vi "DSF.Shared.Configuration.Framework.Convert.From JSON Cluster.vi"(8 "error in (no error)":errorcluster, 10 "Framework Config (JSON)":T1, 11 "Framework Configuration in":refnum<class "DSF.Shared.Configuration.Framework.lvclass">) -> (0 "error out":errorcluster, 3 "Framework Configuration out":refnum<class "DSF.Shared.Configuration.Framework.lvclass">)   [LabVIEW 2017, in "DSF.Engine.lvlib" / "DSF.Shared.Configuration.Framework.lvclass"]
uses:
  DSF.Shared.Configuration.Framework.lvclass
  Typedefs/DELETE.DSF Framework Configuration.ctl
  Typedefs/DELETE.DSF Plugin Configuration.ctl
  DSF Configuration API/1.0.0/Public/Controls/DSF Timing Info.ctl
  Typedefs/DELETE.DSF Transfer Group Configuration.ctl
  Typedefs/DELETE.DSF.Shared.Refactor.Typedefs.JSON.Transfer Configuration.ctl
  DSF Configuration API/1.0.0/Public/Controls/DSF Byte Order.ctl
  Typedefs/DELETE.DSF.Shared.Refactor.Typedefs.JSON.Channel Array Configuration.ctl
  DSF Configuration API/1.0.0/Public/Controls/DSF Settings Info.ctl
  DSF.Shared.Configuration.Framework.lvclass/DSF.Shared.Configuration.Framework.ctl
  DSF.Engine.lvlib
  DSF Configuration API/1.0.0/DSF Configuration API.lvlib
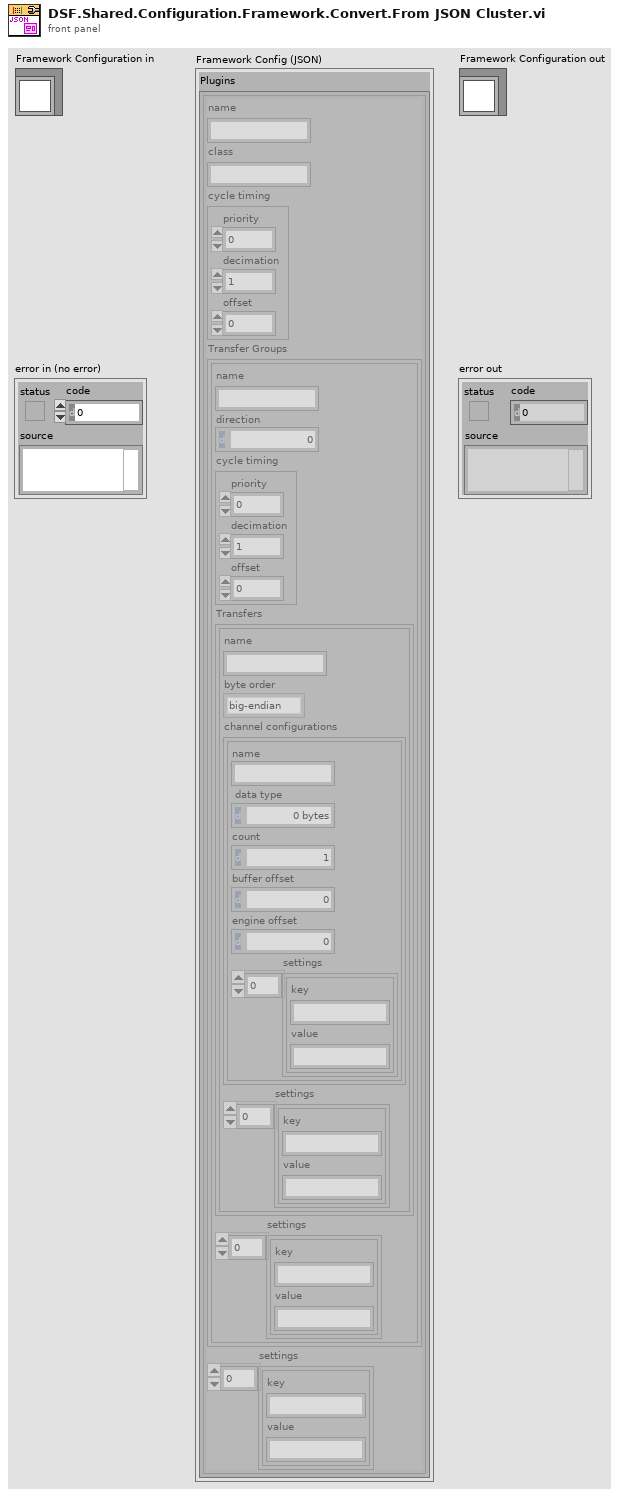
[diagram p1: front panel]
types:
  T1 = typedef "DSF.Engine.lvlib/DELETE.DSF Framework Configuration.ctl" = cluster{"Plugins":T2[]}
  T2 = typedef "DSF.Engine.lvlib/DELETE.DSF Plugin Configuration.ctl" = cluster{"name":string, "class":string, "cycle timing":T3, "Transfer Groups":T4[], "settings":T8}
  T3 = typedef "DSF Configuration API.lvlib/DSF Timing Info.ctl" = cluster{"priority":i32, "decimation":i32, "offset":i32}
  T4 = typedef "DSF.Engine.lvlib/DELETE.DSF Transfer Group Configuration.ctl" = cluster{"name":string, "direction":u8, "cycle timing":T3, "Transfers":T5[], "settings":T8}
  T5 = typedef "DSF.Engine.lvlib/DELETE.DSF.Shared.Refactor.Typedefs.JSON.Transfer Configuration.ctl" = cluster{"name":string, "byte order":T6, "channel configurations":T7[], "settings":T8}
  T6 = typedef "DSF Configuration API.lvlib/DSF Byte Order.ctl" = enum8{"big-endian", "little-endian"}
  T7 = typedef "DSF.Engine.lvlib/DELETE.DSF.Shared.Refactor.Typedefs.JSON.Channel Array Configuration.ctl" = cluster{"name":string, "data type":u8, "count":u64, "buffer offset":u64, "engine offset":u64, "settings":T8}
  T8 = typedef "DSF Configuration API.lvlib/DSF Settings Info.ctl" = cluster{"key":string, "value":string}[]
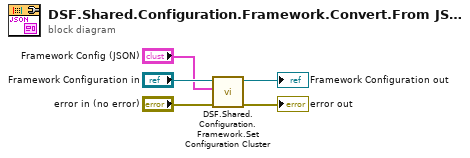
[diagram p0: block diagram]
diagram:
  n1 = call "DSF.Shared.Configuration.Framework.Set Configuration Cluster.vi"("Framework Configuration"="Framework Config (JSON)", "Framework Configuration in"="Framework Configuration in") -> ("Framework Configuration out"=→"Framework Configuration out":refnum<class "DSF.Shared.Configuration.Framework.lvclass">)  [unwired: 9 in]
  "error out" <- "error in (no error)"
